vi "RFSW Get SN List.vi"(8 "Error_In":errorcluster) -> (0 "Error_Out":errorcluster, 1 "SN_Array":string[](array[string]), 2 "Num_Switches":i32, 4 "SN_String":string)   [LabVIEW 2020]
uses:
  C:/Projects/Github/LabVIEW-Tools/Mini-Circuits-RF-Switch/DLL/mcl_RF_Switch_Controller64.dll
  DLL/mcl_RF_Switch_Controller64.dll
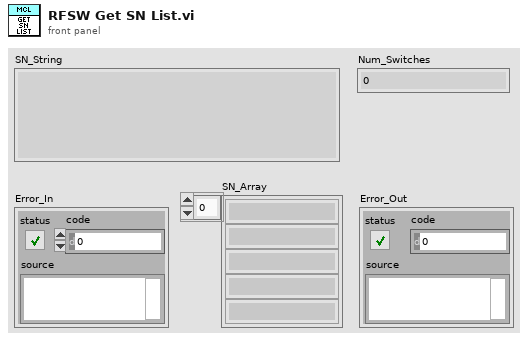
[diagram p1: front panel]
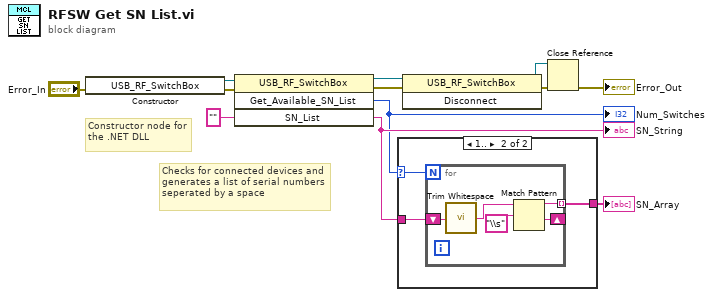
[diagram p0: block diagram]
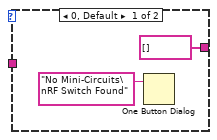
[diagram p2: hidden frame]
diagram:
  # "Checks for connected devices and generates a list of serial numbers seperated by a space"
  # "Constructor node for the .NET DLL"
  n1 = constructor class="USB_RF_SwitchBox"(error in="Error_In") -> (reference out=w10:refnum<k24>, error out=w11:errorcluster)  [unwired: 2 in, 1 out]
  n2 = invoke class="USB_RF_SwitchBox" method="Get_Available_SN_List"(reference=w10, error in=w11, "SN_List"="") -> (reference out=w3:refnum<k24>, error out=w2:errorcluster, "Get_Available_SN_List"=w6:i32, "SN_List"=w8:string)  [unwired: 1 in]
  "SN_String" <- w8
  "Num_Switches" <- w6
  n3 = case shown="1.." w6 {
    selector: w6 -> [_ w15]
    tunnel: w8 -> [_ w17]
    tunnel: [string[] [] w16] -> w7
    frame 0, Default {
      n4 = One Button Dialog(message="No Mini-Circuits\nRF Switch Found") -> ()  [unwired: 1 in, 1 out]
    }
    frame 1.. {
      n5 = for {
        N: w15 -> [_]
        shift-right: [w19] -> _
        shift-left: w17 -> [w22]
        tunnel: [w18] -> w16 mode=indexing
        n6 = call <vilib>:"Trim Whitespace.vi"("string"=w22) -> ("trimmed string"=w21:string)  [unwired: 1 in]
        n7 = Match Pattern(string=w21, regular expression="\\s") -> (before substring=w18:string, after substring=w19:string)  [unwired: 1 in, 2 out]
      }
    }
  }
  "SN_Array" <- w7
  n8 = invoke class="USB_RF_SwitchBox" method="Disconnect"(reference=w3, error in=w2) -> (reference out=w5:refnum<k24>, error out=w4:errorcluster)  [unwired: 1 in, 1 out]
  n9 = Close Reference(reference=w5, error in (no error)=w4) -> (error out=→"Error_Out":errorcluster)
